vi "Cleanup TCP Connection.vi"(8 "error in (no error)":errorcluster, 11 "Websocket Client in":refnum<class "Websocket Client.lvclass">) -> (0 "error out":errorcluster, 3 "Websocket Client out":refnum<class "Websocket Client.lvclass">)   [LabVIEW 2020, in "Stream-Websocket.lvlib" / "Websocket Client.lvclass"]
uses:
  Websocket Client.lvclass
  Websocket Client.lvclass/Websocket Client.ctl
  WebsocketStream/WebsocketStream.lvclass
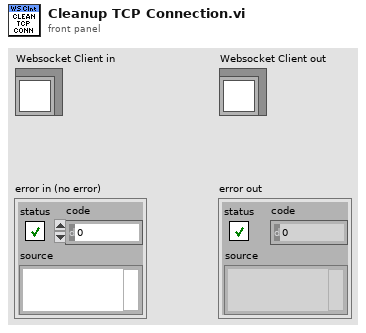
[diagram p1: front panel]
types:
  T1 = typedef "Stream-Websocket.lvlib/Websocket Client.lvclass/Ref Data.ctl" = cluster{"TCP Connection":refnum<k5>, "WS Stream":refnum<class "WebsocketStream.lvclass">, "Connection Loop":refnum<vi>, "Timeout ms":i32, "Server Connection":bool}
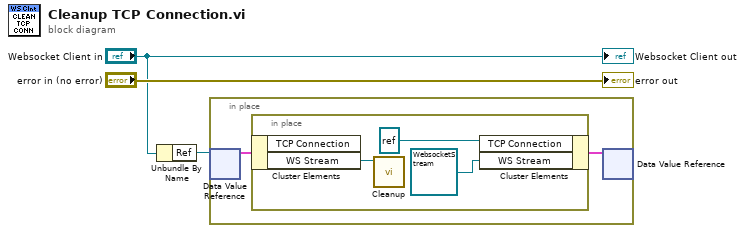
[diagram p0: block diagram]
diagram:
  n1 = Unbundle By Name("Websocket Client in") -> ("Ref"=w2:refnum<data-value>)
  n2 = in-place {
    n3 = in-place-dvr #1(w2) -> (w5:T1)  [unwired: 1 out]
    n4 = in-place {
      n5 = in-place-cluster #2(w5) -> ("WS Stream"=w8:refnum<class "WebsocketStream.lvclass">)  [unwired: 1 out]
      n6 = call "Cleanup.vi"("WebsocketStream in"=w8) -> ()  [unwired: 10 in, 1 out]
      n7 = in-place-cluster #2("TCP Connection"=refnum<k5> refnum, "WS Stream"=refnum<class "WebsocketStream.lvclass"> refnum) -> (w4:T1)
    }
    n8 = in-place-dvr #1(w4) -> ()  [unwired: 2 out]
  }
  "error out" <- "error in (no error)"
  "Websocket Client out" <- "Websocket Client in"
